vi "Modbus Read.vi"(8 "Error In":errorcluster, 10 "Write Buffer":T1={"ID"="\u0001", "Function Code"="\u0003", "Length (High)"="\u0000", "Length (Low)"=",", "Start Address (High)"="\u0000", "Start Address (Middle High)"="\u0000", "Start Address (Middle Low)"="\u0010", "Start Address (Low)"="\u0000", "Data"="\u0000"}, 11 "VISA resource name":refnum<visa-resource-name>) -> (0 "Error Out":errorcluster, 2 "Read Data":string, 3 "VISA resource name out":refnum<visa-resource-name>)   [LabVIEW 2013]
panel:
  out "CRC":string
  out "read buffer":string
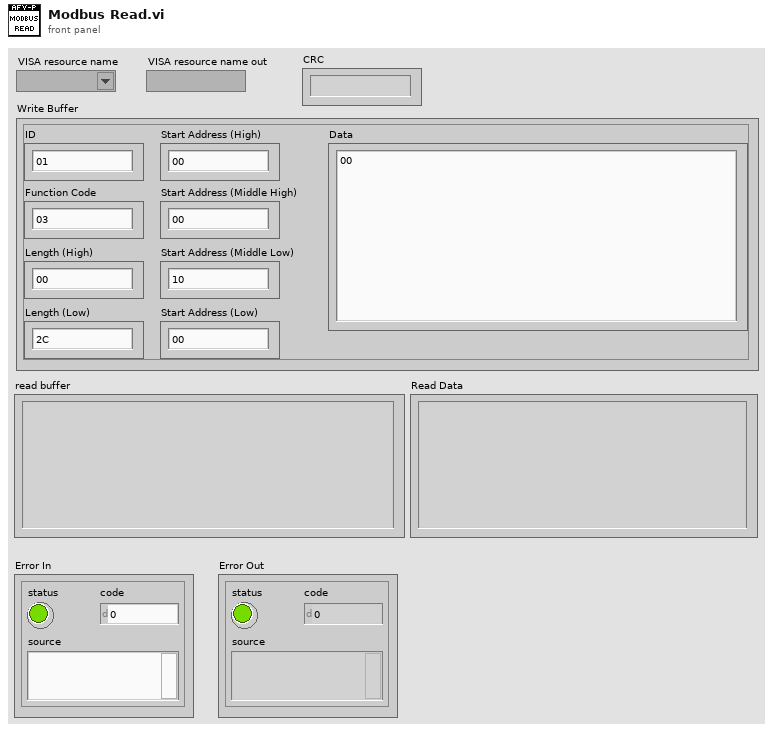
[diagram p1: front panel]
types:
  T1 = cluster{"ID":string, "Function Code":string, "Length (High)":string, "Length (Low)":string, "Start Address (High)":string, "Start Address (Middle High)":string, "Start Address (Middle Low)":string, "Start Address (Low)":string, "Data":string}
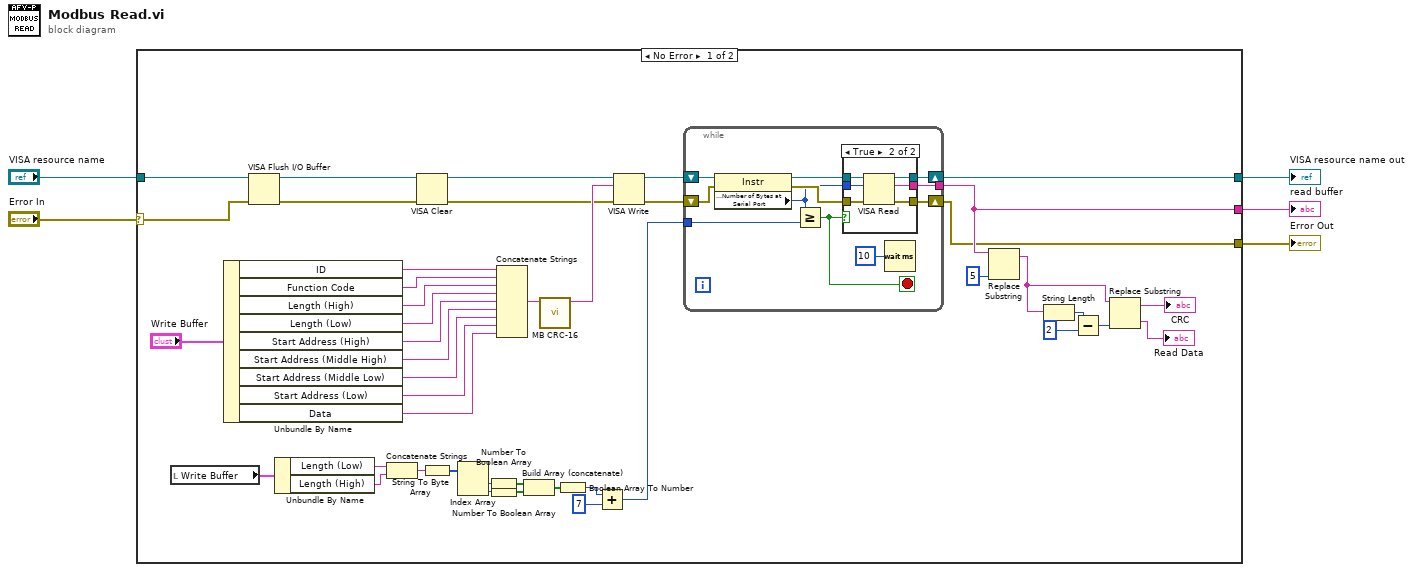
[diagram p0: block diagram]
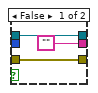
[diagram p2: hidden frame]
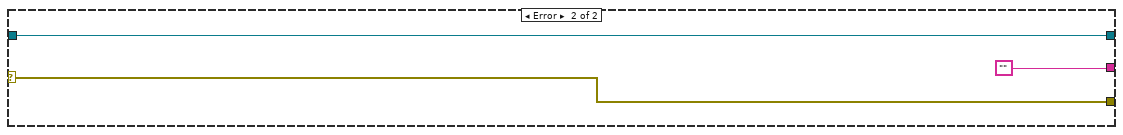
[diagram p3: hidden frame]
diagram:
  n1 = case shown="No Error" "Error In" {
    selector: "Error In" -> [w10 w71]
    tunnel: [w14 ""] -> w5
    tunnel: [w13 w71] -> w3
    tunnel: "VISA resource name" -> [w11 w69]
    tunnel: [w12 w69] -> w1
    frame No Error {
      n2 = local read "Write Buffer"() -> (w22:T1)
      n3 = Unbundle By Name("Write Buffer") -> ("ID"=w42:string, "Function Code"=w38:string, "Length (High)"=w43:string, "Length (Low)"=w44:string, "Start Address (High)"=w45:string, "Start Address (Middle High)"=w46:string, "Start Address (Middle Low)"=w47:string, "Start Address (Low)"=w48:string, "Data"=w39:string)
      n4 = VISA Flush I/O Buffer(VISA resource name=w11, error in (no error)=w10) -> (VISA resource name out=w9:refnum<visa-resource-name>, error out=w8:errorcluster)  [unwired: 1 in]
      n5 = Unbundle By Name(w22) -> ("Length (Low)"=w33:string, "Length (High)"=w34:string)
      n6 = Concatenate Strings(w33, w34) -> (w24:string)
      n7 = VISA Clear(VISA resource name=w9, error in (no error)=w8) -> (VISA resource name out=w6:refnum<visa-resource-name>, error out=w7:errorcluster)
      n8 = String To Byte Array(string=w24) -> (unsigned byte array=w25:u8[])
      n9 = Index Array(array=w25) -> (element #1=w26:u8, element #2=w27:u8)  [unwired: 2 in]
      n10 = Number To Boolean Array(number=w26) -> (Boolean array=w29:bool[])
      n11 = Number To Boolean Array(number=w27) -> (Boolean array=w30:bool[])
      n12 = Concatenate Strings(w42, w38, w43, w44, w45, w46, w47, w48, w39) -> (w40:string)
      n13 = Build Array (concatenate)(w29, w30) -> (w28:bool[])
      n14 = call "MB CRC-16.vi"("String"=w40) -> ("String & CRC-16"=w37:string)  [unwired: 8 in, 2 out]
      n15 = Boolean Array To Number(Boolean array=w28) -> (number=w31:u32)
      n16 = Add(x=w31, y=u32 7) -> (x+y=w23:u32)
      n17 = VISA Write(VISA resource name=w6, write buffer=w37, error in (no error)=w7) -> (VISA resource name out=w35:refnum<visa-resource-name>, error out=w36:errorcluster)  [unwired: 1 out]
      n18 = while {
        tunnel: [w56] -> w14
        tunnel: w23 -> [w55]
        shift-right: [w52] -> w12
        shift-left: w35 -> [w54]
        shift-right: [w51] -> w13
        shift-left: w36 -> [w53]
        stop <- w49 stop-if-true
        n19 = property class="Instr"(reference=w54, error in=w53) -> (reference out=w58:refnum<visa-resource-name>, error out=w57:errorcluster, "Serial Settings:Number of Bytes at Serial Port"=w50:u32)
        n20 = Greater Or Equal?(x=w50, y=w55) -> (x >= y?=w49:bool)
        n21 = case shown="True" w49 {
          tunnel: w58 -> [w61 w68]
          tunnel: w57 -> [w60 w67]
          tunnel: w50 -> [_ w66]
          tunnel: ["" w65] -> w56
          tunnel: [w61 w64] -> w52
          tunnel: [w60 w63] -> w51
          frame False {
          }
          frame True {
            n22 = VISA Read(VISA resource name=w68, byte count=w66, error in (no error)=w67) -> (VISA resource name out=w64:refnum<visa-resource-name>, read buffer=w65:string, error out=w63:errorcluster)  [unwired: 1 out]
          }
        }
        n23 = Wait (ms)(milliseconds to wait=u32 10) -> ()  [unwired: 1 out]
      }
      n24 = Replace Substring(2:5 ("length (len. of substring)"), 5:w14) -> (1:w16:string)  [unwired: 2 in, 1 out]
      n25 = String Length(string=w16) -> (length=w18:i32)
      n26 = Subtract(x=w18, y=2) -> (x-y=w15:i32)
      n27 = Replace Substring(2:w15, 5:w16) -> (0:→"Read Data":string, 1:→"CRC":string)  [unwired: 2 in]
    }
    frame Error {
    }
  }
  "read buffer" <- w5
  "Error Out" <- w3
  "VISA resource name out" <- w1
